vi "report_FGV.vi"(7 "report_mods":T1, 8 "Error In":errorcluster, 10 "Append?":bool, 11 "Data in":variant) -> (0 "Error Out":errorcluster)   [LabVIEW 2016]
uses:
  report_mods.ctl
  report_data.ctl
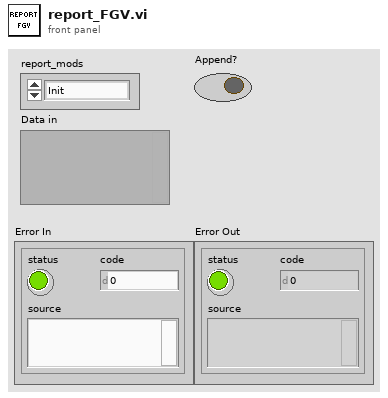
[diagram p1: front panel]
types:
  T1 = typedef "report_mods.ctl" = enum16{"Init", "Table", "Graph", "TablefromGraph", "End"}
  T2 = typedef "report_data.ctl" = cluster{"FileData":refnum<file>, "FileAppend":refnum<file>, "PathData":path, "PathAppend":path}
  T3 = enum16{"open", "replace", "create", "open or create", "replace or create", "replace or create with confirmation"}
  T4 = cluster{string, "reference":refnum<vi>, "string":string[]}
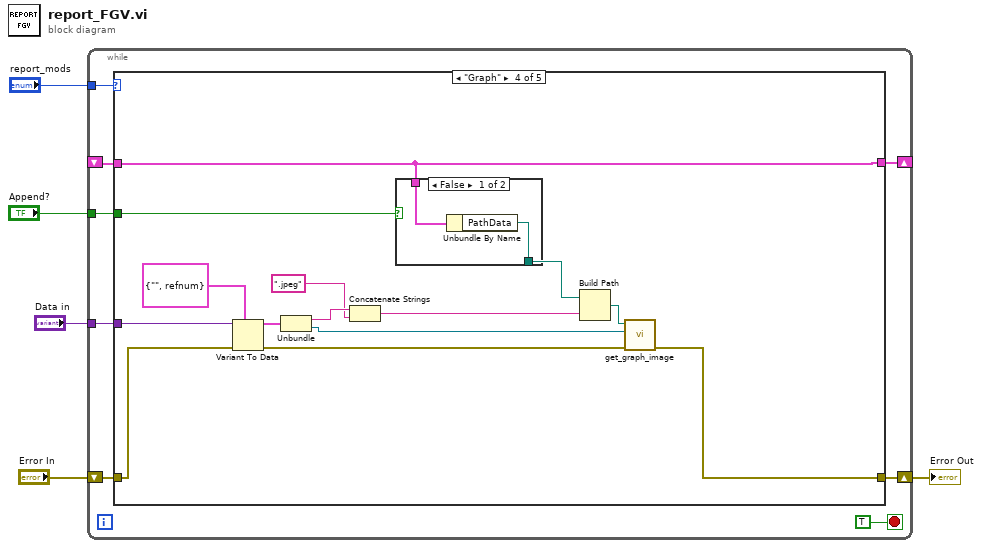
[diagram p0: block diagram]
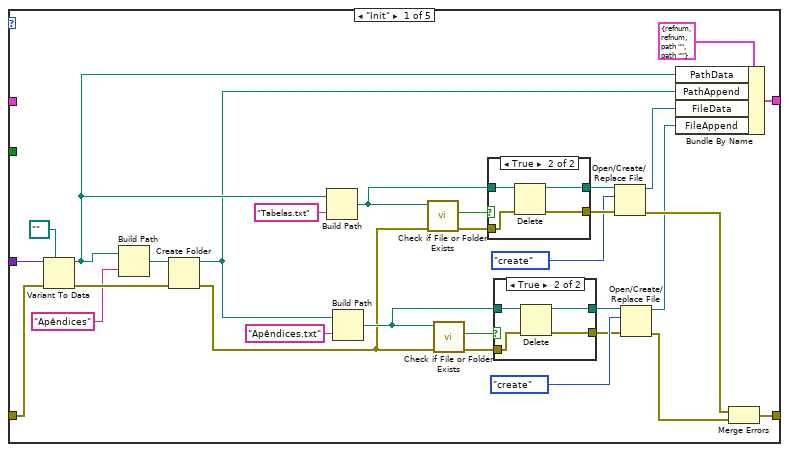
[diagram p2: hidden frame]
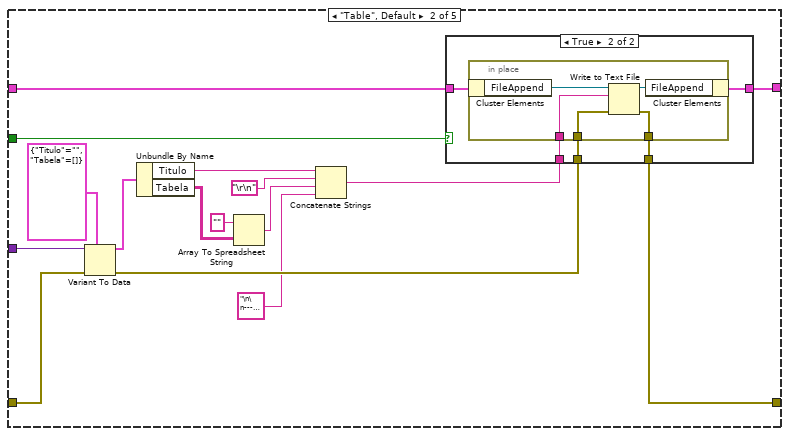
[diagram p5: hidden frame]
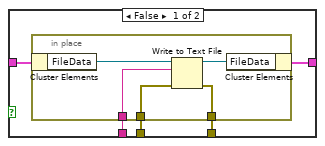
[diagram p6: hidden frame]
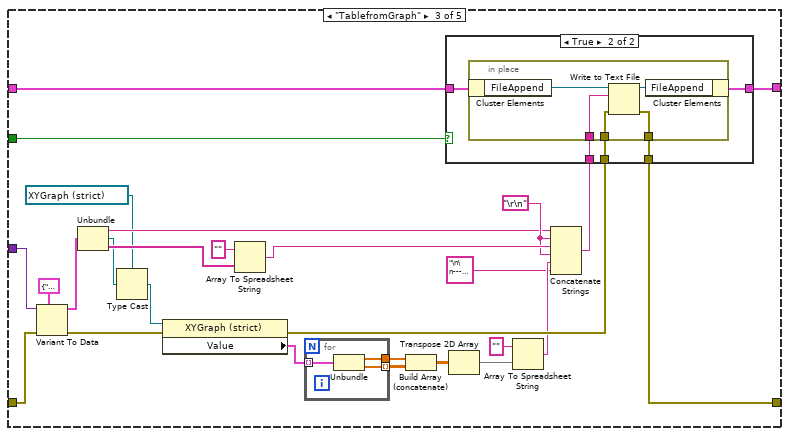
[diagram p7: hidden frame]
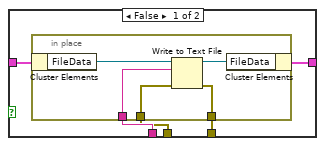
[diagram p8: hidden frame]
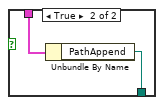
[diagram p9: hidden frame]
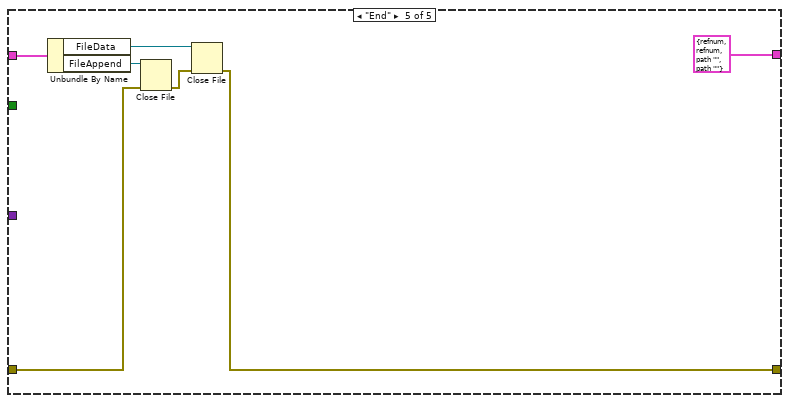
[diagram p10: hidden frame]
diagram:
  n1 = while {
    tunnel: "report_mods" -> [w13]
    shift-right: [w10] -> w3
    shift-left: "Error In" -> [w11]
    tunnel: "Data in" -> [w9]
    shift-right: [w8] -> _
    shift-left: _ -> [w6]
    tunnel: "Append?" -> [w7]
    stop <- TRUE stop-if-true
    n2 = case shown="\"Graph\"" w13 {
      tunnel: w11 -> [w25 w67 w114 w152 w164]
      tunnel: [w27 w69 w116 w144 w162] -> w10
      tunnel: w9 -> [w26 w68 w115 w153 _]
      tunnel: [w14 w64 w112 w141 T2 {"FileData"=refnum, "FileAppend"=refnum, "PathData"=path "", "PathAppend"=path ""} ("report_data")] -> w8
      tunnel: w7 -> [_ w63 w111 w142 _]
      tunnel: w6 -> [_ w65 w113 w141 w160]
      frame "Init" {
        n3 = Variant To Data(error in=w25, type=path "", Variant=w26) -> (data=w18:path, error out=w23:errorcluster)
        n4 = Build Path(base path=w18, name or relative path="Apêndices") -> (appended path=w20:path)
        n5 = Create Folder(path (use dialog)=w20, error in=w23) -> (created path=w17:path, error out=w22:errorcluster)  [unwired: 1 in, 1 out]
        n6 = Build Path(base path=w18, name or relative path="Tabelas.txt") -> (appended path=w41:path)
        n7 = Build Path(base path=w17, name or relative path="Apêndices.txt") -> (appended path=w34:path)
        n8 = call <vilib>:"Check if File or Folder Exists.vi"("error in (no error)"=w22, "path"=w41) -> ("error out"=w31:errorcluster, "file or folder exists?"=w42:bool)  [unwired: 7 in, 1 out]
        n9 = call <vilib>:"Check if File or Folder Exists.vi"("error in (no error)"=w22, "path"=w34) -> ("error out"=w30:errorcluster, "file or folder exists?"=w33:bool)  [unwired: 7 in, 1 out]
        n10 = case shown="True" w42 {
          tunnel: w41 -> [w49 w53]
          tunnel: [_ w52] -> w40
          tunnel: [w49 w51] -> w39
          tunnel: w31 -> [_ w50]
          frame False {
          }
          frame True {
            n11 = Delete(path (use dialog)=w53, error in=w50) -> (deleted path=w51:path, error out=w52:errorcluster)  [unwired: 3 in, 1 out]
          }
        }
        n12 = case shown="True" w33 {
          tunnel: w34 -> [w44 w48]
          tunnel: [_ w47] -> w35
          tunnel: [w44 w46] -> w36
          tunnel: w30 -> [_ w45]
          frame False {
          }
          frame True {
            n13 = Delete(path (use dialog)=w48, error in=w45) -> (deleted path=w46:path, error out=w47:errorcluster)  [unwired: 3 in, 1 out]
          }
        }
        n14 = Open/Create/Replace File(file path (use dialog)=w39, error in=w40, operation (0:open)=T3."create") -> (refnum out=w16:refnum<file>, error out=w28:errorcluster)  [unwired: 3 in, 1 out]
        n15 = Open/Create/Replace File(file path (use dialog)=w36, error in=w35, operation (0:open)=T3."create") -> (refnum out=w15:refnum<file>, error out=w29:errorcluster)  [unwired: 3 in, 1 out]
        n16 = Bundle By Name(cluster=T2 {"FileData"=refnum, "FileAppend"=refnum, "PathData"=path "", "PathAppend"=path ""} ("report_data"), "PathData"=w18, "PathAppend"=w17, "FileData"=w16, "FileAppend"=w15) -> (w14:T2)
        n17 = Merge Errors(w28, w29) -> (w27:errorcluster)
      }
      frame "Table", Default {
        n18 = Variant To Data(error in=w67, type=cluster{"Titulo":string, "Tabela":string[][]} {"Titulo"="", "Tabela"=[]}, Variant=w68) -> (data=w60:cluster{"Titulo":string, "Tabela":string[][]}, error out=w66:errorcluster)
        n19 = Unbundle By Name(w60) -> ("Titulo"=w57:string, "Tabela"=w59:string[][])
        n20 = Array To Spreadsheet String(array=w59, 3:"" ("format string")) -> (spreadsheet string=w55:string)  [unwired: 1 in]
        n21 = Concatenate Strings(w57, "\r\n", w55, "\n\n---   ---   ---   ---   ---   ---   ---   ---   ---   ---   \n\n" ("string")) -> (w62:string)
        n22 = case shown="True" w63 {
          tunnel: [w74 w84] -> w69
          tunnel: w62 -> [w73 w83]
          tunnel: w66 -> [w72 w82]
          tunnel: w65 -> [w71 w81]
          tunnel: [w70 w80] -> w64
          frame False {
            n23 = in-place {
              in-place-border: [w79] -> w74
              in-place-border: w73 -> [w78]
              in-place-border: w72 -> [w77]
              n24 = in-place-cluster #1(w71) -> ("FileData"=w76:refnum<file>)
              n25 = Write to Text File(file (use dialog)=w76, text=w78, error in=w77) -> (refnum out=w75:refnum<file>, error out=w79:errorcluster)  [unwired: 1 in, 1 out]
              n26 = in-place-cluster #1("FileData"=w75) -> (w70:T2)
            }
          }
          frame True {
            n27 = in-place {
              in-place-border: [w89] -> w84
              in-place-border: w83 -> [w88]
              in-place-border: w82 -> [w87]
              n28 = in-place-cluster #2(w81) -> ("FileAppend"=w86:refnum<file>)
              n29 = Write to Text File(file (use dialog)=w86, text=w88, error in=w87) -> (refnum out=w85:refnum<file>, error out=w89:errorcluster)  [unwired: 1 in, 1 out]
              n30 = in-place-cluster #2("FileAppend"=w85) -> (w80:T2)
            }
          }
        }
      }
      frame "TablefromGraph" {
        w107 = "\r\n"
        n31 = Variant To Data(error in=w114, type=T4 {"", "reference"=refnum, "string"=[]} ("output cluster"), Variant=w115) -> (data=w97:T4, error out=w93:errorcluster)
        n32 = Unbundle(w97) -> (w96:string, "reference"=w92:refnum<vi>, "string"=w95:string[])
        n33 = Type Cast(type=refnum<vi> refnum ("Stress"), x=w92) -> (*(type *) &x=w90:refnum<vi>)
        n34 = property class="XYGraph (strict)"(reference=w90, error in=w93) -> (error out=w103:errorcluster, "Value"=w106:cluster{"z":dbl[], dbl[]}[])  [unwired: 1 out]
        n35 = Array To Spreadsheet String(array=w95, 3:"" ("format string")) -> (spreadsheet string=w108:string)  [unwired: 1 in]
        n36 = for {
          tunnel: w106 -> [w119] mode=indexing
          tunnel: [w118] -> w105 mode=indexing
          tunnel: [w117] -> w104
          n37 = Unbundle(w119) -> ("z"=w117:dbl[], w118:dbl[])
        }
        n38 = Build Array (concatenate)(w104, w105) -> (w102:dbl[][])
        n39 = Transpose 2D Array(2D array=w102) -> (transposed array=w100:dbl[][])
        n40 = Array To Spreadsheet String(array=w100, 3:"" ("format string")) -> (spreadsheet string=w99:string)  [unwired: 1 in]
        n41 = Concatenate Strings(w96, w107, w108, w107, w99, "\n\n---   ---   ---   ---   ---   ---   ---   ---   ---   ---   \n\n" ("string")) -> (w110:string)
        n42 = case shown="True" w111 {
          tunnel: [w124 w134] -> w116
          tunnel: w110 -> [w123 w133]
          tunnel: w103 -> [w122 w132]
          tunnel: w113 -> [w121 w131]
          tunnel: [w120 w130] -> w112
          frame False {
            n43 = in-place {
              in-place-border: [w129] -> w124
              in-place-border: w123 -> [w128]
              in-place-border: w122 -> [w127]
              n44 = in-place-cluster #3(w121) -> ("FileData"=w126:refnum<file>)
              n45 = Write to Text File(file (use dialog)=w126, text=w128, error in=w127) -> (refnum out=w125:refnum<file>, error out=w129:errorcluster)  [unwired: 1 in, 1 out]
              n46 = in-place-cluster #3("FileData"=w125) -> (w120:T2)
            }
          }
          frame True {
            n47 = in-place {
              in-place-border: [w139] -> w134
              in-place-border: w133 -> [w138]
              in-place-border: w132 -> [w137]
              n48 = in-place-cluster #4(w131) -> ("FileAppend"=w136:refnum<file>)
              n49 = Write to Text File(file (use dialog)=w136, text=w138, error in=w137) -> (refnum out=w135:refnum<file>, error out=w139:errorcluster)  [unwired: 1 in, 1 out]
              n50 = in-place-cluster #4("FileAppend"=w135) -> (w130:T2)
            }
          }
        }
      }
      frame "Graph" {
        n51 = Variant To Data(error in=w152, type=cluster{string, "reference":refnum<vi>} {"", "reference"=refnum}, Variant=w153) -> (data=w150:cluster{string, "reference":refnum<vi>}, error out=w149:errorcluster)
        n52 = Unbundle(w150) -> (w148:string, "reference"=w143:refnum<vi>)
        n53 = Concatenate Strings(w148, ".jpeg" ("string")) -> (w146:string)
        n54 = case shown="False" w142 {
          tunnel: w141 -> [w155 w157]
          tunnel: [w154 w156] -> w140
          frame False {
            n55 = Unbundle By Name(w155) -> ("PathData"=w154:path)
          }
          frame True {
            n56 = Unbundle By Name(w157) -> ("PathAppend"=w156:path)
          }
        }
        n57 = Build Path(base path=w140, name or relative path=w146) -> (appended path=w145:path)
        n58 = call "get_graph_image.vi"("error in"=w149, "reference"=w143, "Path"=w145) -> ("error out"=w144:errorcluster)  [unwired: 8 in]
      }
      frame "End" {
        n59 = Unbundle By Name(w160) -> ("FileData"=w158:refnum<file>, "FileAppend"=w159:refnum<file>)
        n60 = Close File(refnum=w159, error in=w164) -> (error out=w163:errorcluster)  [unwired: 1 out]
        n61 = Close File(refnum=w158, error in=w163) -> (error out=w162:errorcluster)  [unwired: 1 out]
      }
    }
  }
  "Error Out" <- w3
